vi "Set Edge Trigger.vi"(6 "Trigger Slope (0: Rising)":u16(ring) items=["Rising", "Falling", "Either"], 7 "Trigger Coupling (0 : DC)":u16(ring) items=["DC", "HF Reject", "LF Reject", "Noise Reject", "AC"], 8 "error in (no error)":errorcluster, 9 "Trigger Level (0.0 V)":dbl, 10 "Analog Channel":T1, 11 "PXIe5105 in":refnum<class "PXIe5105.lvclass">) -> (0 "error out":errorcluster, 3 "PXIe5105 out":refnum<class "PXIe5105.lvclass">)   [LabVIEW 2018, in "PXIe5105.lvlib" / "PXIe5105.lvclass"]
uses:
  PXIe5105.lvclass
  PPLs/Oscilloscope/Parent/Oscilloscope.lvlibp/Custom Controls/Analog Channels.ctl
  <instrlib>/niScope/Controls/niScope trigger slope.ctl
  <instrlib>/niScope/Controls/niScope trigger coupling.ctl
  PXIe5105.lvclass/PXIe5105.ctl
  <instrlib>/niScope/Configure/Trigger/niScope Configure Trigger Edge.vi
  PPLs/Oscilloscope/Parent/Oscilloscope.lvlibp
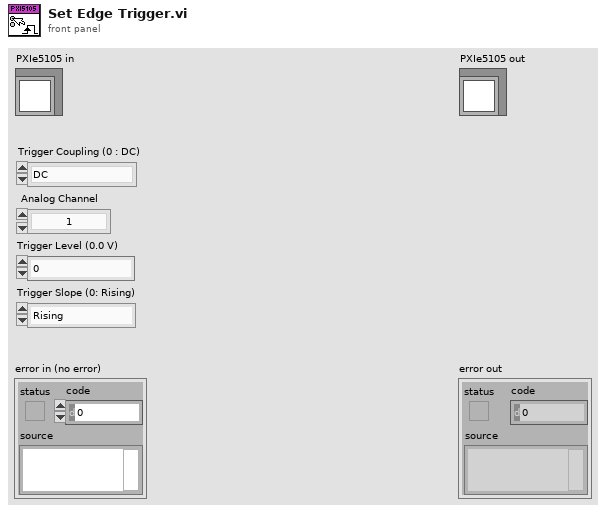
[diagram p1: front panel]
types:
  T1 = typedef "Oscilloscope.lvlibp/Analog Channels.ctl" = enum16{"1", "2", "3", "4", "5", "6", "7", "8", "9", "10", "11", "12", "13", "14", "15", "16"}
  T2 = typedef "niScope trigger coupling.ctl" = u16
  T3 = typedef "niScope trigger slope.ctl" = i32
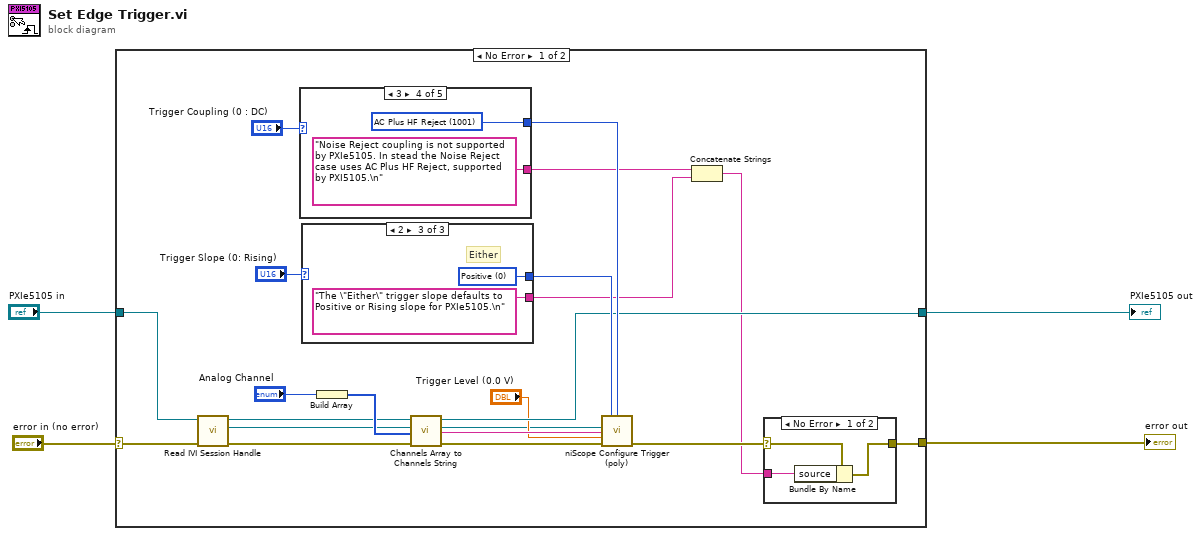
[diagram p0: block diagram]
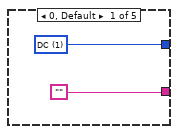
[diagram p3: hidden frame]
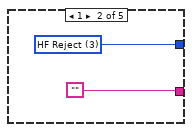
[diagram p4: hidden frame]
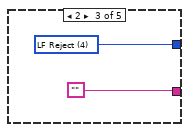
[diagram p5: hidden frame]
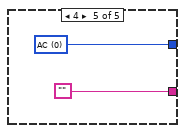
[diagram p6: hidden frame]
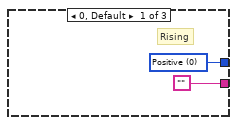
[diagram p7: hidden frame]
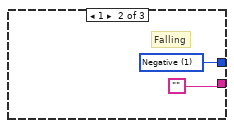
[diagram p8: hidden frame]
diagram:
  n1 = case shown="No Error" "error in (no error)" {
    selector: "error in (no error)" -> [w8 w46]
    tunnel: [w10 w46] -> w3
    tunnel: [w17 w45] -> w2
    tunnel: "PXIe5105 in" -> [w9 w45]
    frame No Error {
      n2 = call "Read IVI Session Handle.vi"("error in (no error)"=w8, "PXIe5105 in"=w9) -> ("error out"=w6:errorcluster, "IVI Session Handle"=w5:refnum<k15>, "PXIe5105 out"=w7:refnum<class "PXIe5105.lvclass">)  [unwired: 7 in]
      n3 = case shown="3" "Trigger Coupling (0 : DC)" {
        tunnel: [w30 w32 w34 w36 w38] -> w21
        tunnel: ["" "" "" "Noise Reject coupling is not supported by PXIe5105. In stead the Noise Reject case uses AC Plus HF Reject, supported by PXI5105.\n" ""] -> w13
        frame 0, Default {
          w30 = T2 1 items=["AC"=0, "DC"=1, "HF Reject"=3, "LF Reject"=4, "AC Plus HF Reject"=1001] ("trigger coupling")
        }
        frame 1 {
          w32 = T2 3 items=["AC"=0, "DC"=1, "HF Reject"=3, "LF Reject"=4, "AC Plus HF Reject"=1001] ("trigger coupling")
        }
        frame 2 {
          w34 = T2 4 items=["AC"=0, "DC"=1, "HF Reject"=3, "LF Reject"=4, "AC Plus HF Reject"=1001] ("trigger coupling")
        }
        frame 3 {
          w36 = T2 1001 items=["AC"=0, "DC"=1, "HF Reject"=3, "LF Reject"=4, "AC Plus HF Reject"=1001] ("trigger coupling")
        }
        frame 4 {
          w38 = T2 0 items=["AC"=0, "DC"=1, "HF Reject"=3, "LF Reject"=4, "AC Plus HF Reject"=1001] ("trigger coupling")
        }
      }
      n4 = case shown="2" "Trigger Slope (0: Rising)" {
        tunnel: [w40 w42 w44] -> w24
        tunnel: ["" "" "The \"Either\" trigger slope defaults to Positive or Rising slope for PXIe5105.\n"] -> w12
        frame 0, Default {
          w40 = T3 0 items=["Positive", "Negative"] ("trigger slope")
          # "Rising"
        }
        frame 1 {
          w42 = T3 1 items=["Positive", "Negative"] ("trigger slope")
          # "Falling"
        }
        frame 2 {
          w44 = T3 0 items=["Positive", "Negative"] ("trigger slope")
          # "Either"
        }
      }
      n5 = Build Array("Analog Channel") -> (w19:T1[])
      n6 = call "Channels Array to Channels String.vi"("error in (no error)"=w6, "Channel(s) Array"=w19, "PXIe5105 in"=w7) -> ("error out"=w15:errorcluster, "Channels String"=w18:string, "PXIe5105 out"=w17:refnum<class "PXIe5105.lvclass">)  [unwired: 6 in]
      n7 = call-poly <instrlib>:"niScope Configure Trigger (poly).vi"("instrument handle"=w5, "trigger slope"=w24, "trigger coupling"=w21, "trigger source"=w18, "trigger level"="Trigger Level (0.0 V)", "error in"=w15) -> ("error out"=w14:errorcluster)  [unwired: 8 in, 1 out]
      n8 = Concatenate Strings(w13, w12) -> (w11:string)
      n9 = case shown="No Error" w14 {
        selector: w14 -> [w27 w28]
        tunnel: w11 -> [w26 _]
        tunnel: [w25 w28] -> w10
        frame No Error {
          n10 = Bundle By Name(cluster=w27, "source"=w26) -> (w25:errorcluster)
        }
        frame Error {
        }
      }
    }
    frame Error {
    }
  }
  "error out" <- w3
  "PXIe5105 out" <- w2
